vi "Open Device.vi"(8 "error in (no error)":errorcluster, 9 "_Serial Number":string, 10 "Config File":path, 11 "Topas in":refnum<class "Topas3.lvclass">) -> (0 "error out":errorcluster, 3 "Topas out":refnum<class "Topas3.lvclass">)   [LabVIEW 2020, in "Topas3.lvclass"]
uses:
  Topas3.lvclass
  Topas3.lvclass/Topas3.ctl
  Topas-LabVIEW-Driver/TopasDriver.lvlib
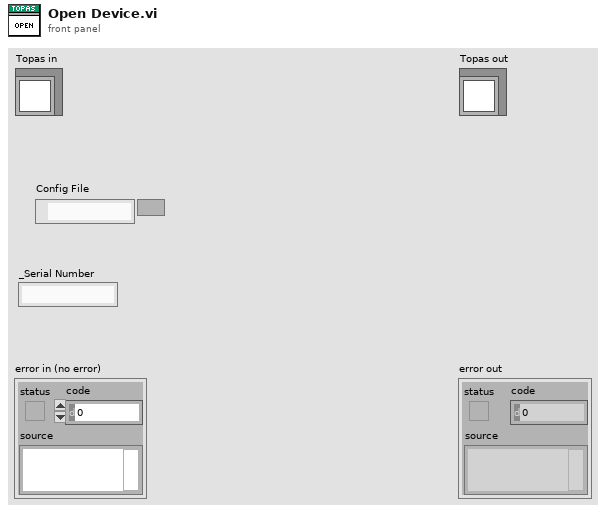
[diagram p1: front panel]
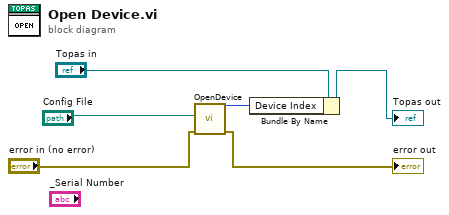
[diagram p0: block diagram]
diagram:
  n1 = call "OpenDevice.vi"("error in (no error)"="error in (no error)", "path"="Config File") -> ("error out"=→"error out":errorcluster, "Device Index"=w1:u8)  [unwired: 8 in]
  n2 = Bundle By Name(cluster="Topas in", "Device Index"=w1) -> (→"Topas out":refnum<class "Topas3.lvclass">)
